vi "Write LVCAM.vi"(10 "LVCAM":refnum<class "LVCAM.lvclass">, 11 "Write LVCAM in":refnum<class "Write LVCAM.lvclass">) -> (3 "Write LVCAM out":refnum<class "Write LVCAM.lvclass">)   [LabVIEW 2021, in "LVCAM.lvlib" / "Write LVCAM.lvclass"]
uses:
  Write LVCAM.lvclass
  LVCAM/LVCAM.lvclass
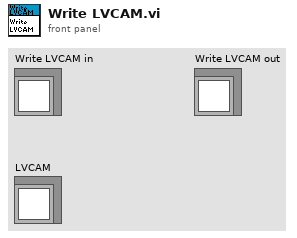
[diagram p1: front panel]
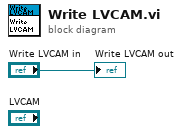
[diagram p0: block diagram]
diagram:
  "Write LVCAM out" <- "Write LVCAM in"
